vi "get_centering.vi"(0 "TrajectoryTS090820Circular2D in":refnum<class "TrajectoryTS090820Circular2D.lvclass">, 5 "error in (no error)":errorcluster) -> (14 "TrajectoryTS090820Circular2D out":refnum<class "TrajectoryTS090820Circular2D.lvclass">, 15 "x center":dbl, 16 "y center":dbl, 17 "z center":dbl, 18 "rotation angle":dbl, 19 "error out":errorcluster)   [LabVIEW 2010, in "TrajectoryTS090820Circular2D.lvclass"]
uses:
  TrajectoryTS090820Circular2D.lvclass
  TrajectoryTS090820Circular2D.lvclass/TrajectoryTS090820Circular2D.ctl
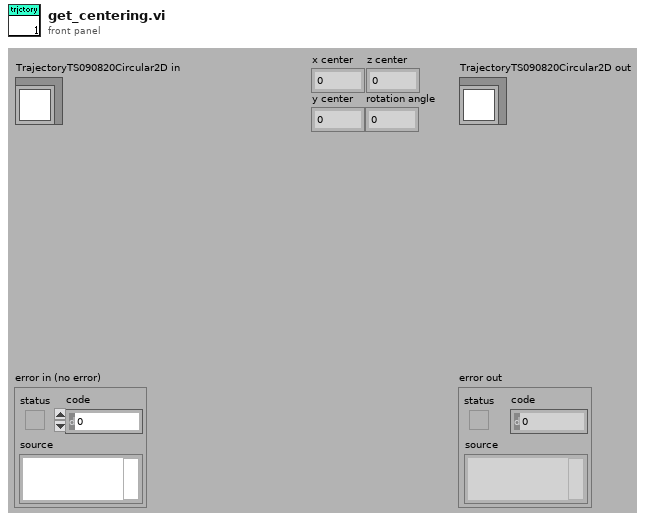
[diagram p1: front panel]
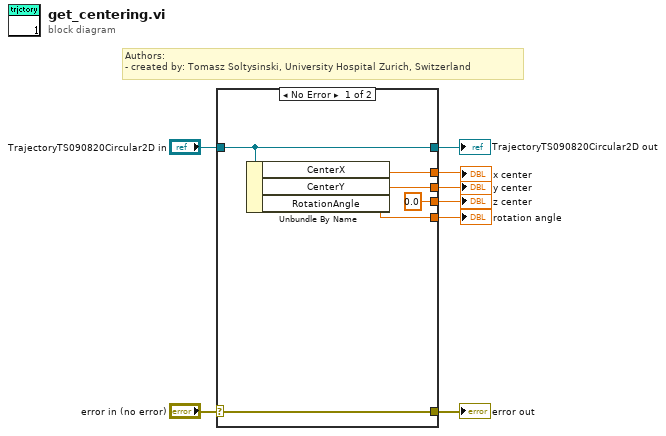
[diagram p0: block diagram]
diagram:
  # "Authors: \n- created by: Tomasz Soltysinski, University Hospital Zurich, Switzerland"
  n1 = case shown="No Error" "error in (no error)" {
    selector: "error in (no error)" -> [w14 w16]
    tunnel: [w14 w16] -> w7
    tunnel: [w13 w15] -> w5
    tunnel: "TrajectoryTS090820Circular2D in" -> [w13 w15]
    tunnel: [w12 _] -> w4
    tunnel: [w11 _] -> w3
    tunnel: [0.0 ("z center") _] -> w2
    tunnel: [w10 _] -> w1
    frame No Error {
      n2 = Unbundle By Name(w13) -> ("CenterX"=w12:dbl, "CenterY"=w11:dbl, "RotationAngle"=w10:dbl)
    }
    frame Error {
    }
  }
  "error out" <- w7
  "TrajectoryTS090820Circular2D out" <- w5
  "x center" <- w4
  "y center" <- w3
  "z center" <- w2
  "rotation angle" <- w1
